vi "ThingworxClose.vi"(3 "error in (no error)":errorcluster, 5 "Thing Info Out":T2) -> (0 "error out":errorcluster)   [LabVIEW 2015]
uses:
  <vilib>/httpClient/ClientHandle.ctl
  <vilib>/httpClient/LabVIEWHTTPClient.lvlib
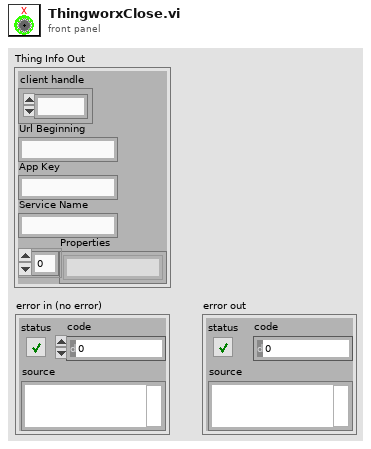
[diagram p1: front panel]
types:
  T1 = typedef "LabVIEWHTTPClient.lvlib/ClientHandle.ctl" = refnum<k1>
  T2 = cluster{"client handle":T1, "Url Beginning":string, "App Key":string, "Service Name":string, "Properties":string[]}
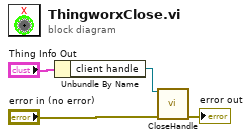
[diagram p0: block diagram]
diagram:
  n1 = Unbundle By Name("Thing Info Out") -> ("client handle"=w4:T1)
  n2 = call <vilib>:"CloseHandle.vi"("client handle"=w4, "error in (no error)"="error in (no error)") -> ("error out"=→"error out":errorcluster)  [unwired: 13 in]
